vi "New Assert Message.vi"(8 "error in (no error)":errorcluster, 10 "Assert Message":T1, 11 "Standard Display Configuration in":refnum<class "Standard Display Configuration.lvclass">) -> (0 "error out":errorcluster, 3 "Standard Display Configuration out":refnum<class "Standard Display Configuration.lvclass">)   [LabVIEW 2016, in "Assert API Components.lvlib" / "Assert Display.lvlib" / "Main Display.lvlib" / "Standard Display Configuration.lvclass"]
uses:
  Standard Display Configuration.lvclass
  D:/Work/Projects/actor_assert_api/Main Display/Display Configurations/Base Display Configuration.lvclass
  Assert API Components/Message Data.ctl
  Assert API Components/VI References.ctl
  Base Display Configuration.lvclass/Base Display Configuration.ctl
  Standard Display Configuration.lvclass/Standard Display Configuration.ctl
  Base Display Configuration.lvclass
  Assert API Components/Assert API Components.lvlib
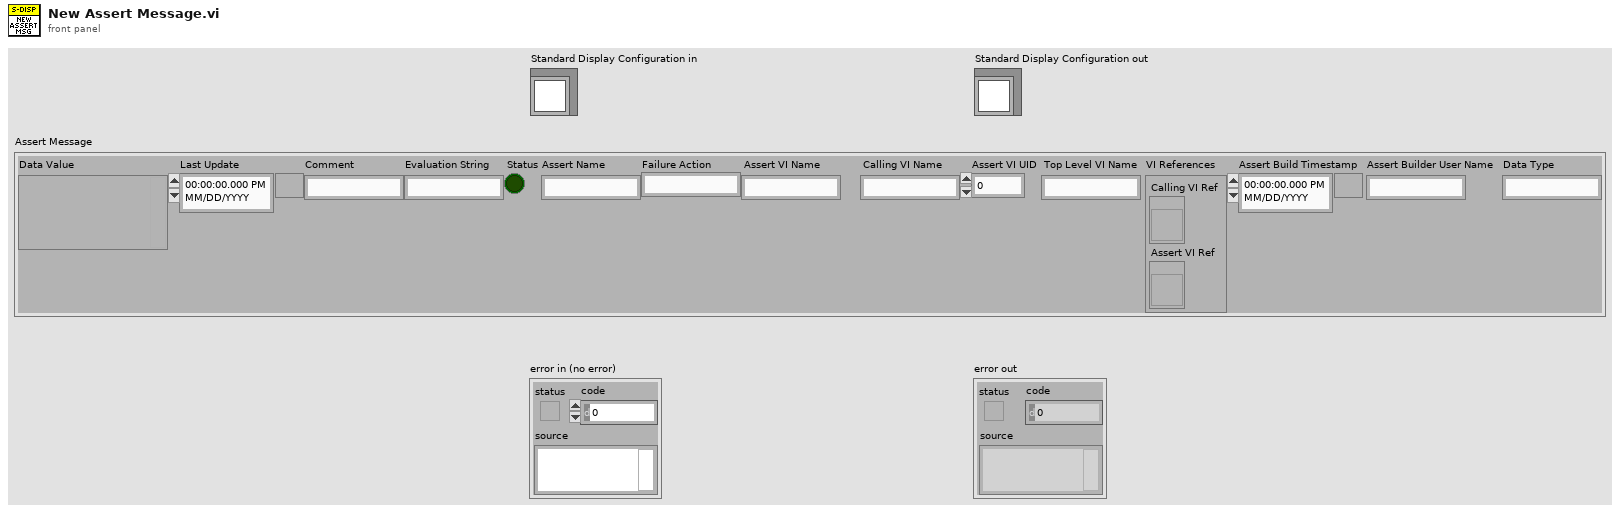
[diagram p1: front panel]
types:
  T1 = typedef "Assert API Components.lvlib/Message Data.ctl" = cluster{"Data Value":variant, "Last Update":timestamp, "Comment":string, "Evaluation String":string, "Status":bool, "Assert Name":string, "Failure Action":string, "Assert VI Name":string, "Calling VI Name":string, "Assert VI UID":i32, "Top Level VI Name":string, "VI References":T2, "Assert Build Timestamp":timestamp, "Assert Builder User Name":string, "Data Type":string}
  T2 = typedef "Assert API Components.lvlib/VI References.ctl" = cluster{"Calling VI Ref":refnum<vi>, "Assert VI Ref":refnum<vi>}
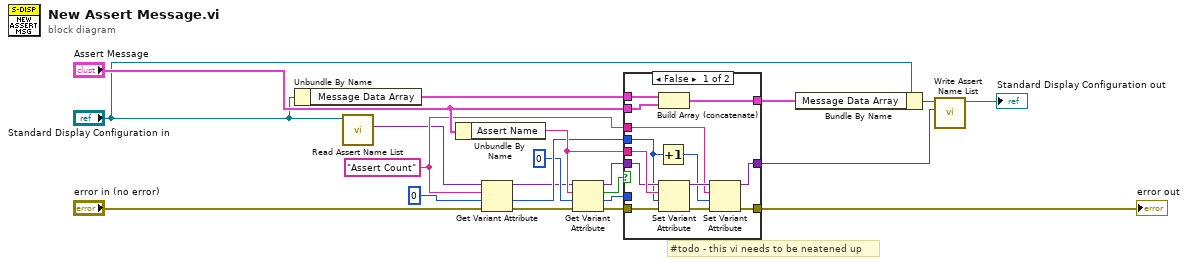
[diagram p0: block diagram]
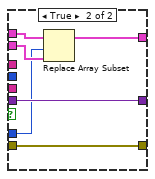
[diagram p2: hidden frame]
diagram:
  w9 = "Assert Count" ("name")
  # "#todo - this vi needs to be neatened up"
  n1 = Unbundle By Name("Standard Display Configuration in") -> ("Message Data Array"=w19:T1[])
  n2 = call "Read Assert Name List.vi"("Base Display Configuration in"="Standard Display Configuration in") -> ("Assert Name List"=w1:variant)  [unwired: 10 in]
  n3 = Unbundle By Name("Assert Message") -> ("Assert Name"=w14:string)
  n4 = Get Variant Attribute(Variant=w1, name=w9, default value (empty Variant)=0, error in="error in (no error)") -> (duplicate Variant=w6:variant, value=w11:i32, error out=w7:errorcluster)  [unwired: 1 out]
  n5 = Get Variant Attribute(Variant=w6, name=w14, default value (empty Variant)=0, error in=w7) -> (duplicate Variant=w13:variant, found=w17:bool, value=w10:i32, error out=w15:errorcluster)
  n6 = case shown="False" w17 {
    tunnel: [w34 w38] -> w20
    tunnel: w19 -> [w33 w40]
    tunnel: "Assert Message" -> [w32 w39]
    tunnel: w11 -> [w22 _]
    tunnel: w15 -> [w31 w36]
    tunnel: w14 -> [w30 _]
    tunnel: w13 -> [w29 w37]
    tunnel: [w25 w37] -> w3
    tunnel: [w27 w36] -> w12
    tunnel: w10 -> [_ w35]
    tunnel: w9 -> [w24 _]
    frame False {
      n7 = Increment(x=w22) -> (x+1=w23:i32)
      n8 = Build Array (concatenate)(w33, w32) -> (w34:T1[])
      n9 = Set Variant Attribute(Variant=w29, name=w30, value=w22, error in=w31) -> (Variant out=w26:variant, error out=w28:errorcluster)  [unwired: 1 out]
      n10 = Set Variant Attribute(Variant=w26, name=w24, value=w23, error in=w28) -> (Variant out=w25:variant, error out=w27:errorcluster)  [unwired: 1 out]
    }
    frame True {
      n11 = Replace Array Subset(array=w40, new element=w39, index=w35) -> (w38:T1[])
    }
  }
  "error out" <- w12
  n12 = Bundle By Name(cluster="Standard Display Configuration in", "Message Data Array"=w20) -> (w21:refnum<class "Standard Display Configuration.lvclass">)
  n13 = call "Write Assert Name List.vi"("Assert Name List"=w3, "Base Display Configuration in"=w21) -> ("Base Display Configuration out"=→"Standard Display Configuration out":refnum<class "Standard Display Configuration.lvclass">)  [unwired: 9 in]
